vi "Execute.vi"(8 "error in (no error)":errorcluster, 9 "write enable":bool=TRUE, 10 "stop":bool, 11 "MB_TCP in":refnum<class "MB_TCP.lvclass">) -> (0 "error out":errorcluster, 2 "stopped":bool, 3 "MB_TCP out":refnum<class "MB_TCP.lvclass">)   [LabVIEW 2021, in "MB_TCP.lvclass"]
uses:
  MB_TCP.lvclass
  MB_TCP_State.ctl
  MB_TCP.lvclass/MB_TCP.ctl
  NI_modbus_upd/TCP/TCP.lvclass/TCP.ctl
  ICPCON Registers/MB ICPCON Registers Write DO.vi
  ICPCON Registers/MB ICPCON Registers Write IR.vi
  ICPCON Registers/MB ICPCON Registers Write DI.vi
  ICPCON Registers/MB ICPCON Registers Write OR.vi
  NI_modbus_upd/TCP/Accessors/Address/Write Address.vi
  NI_modbus_upd/TCP/Accessors/Port/Write Port.vi
  NI_modbus_upd/TCP/Accessors/connect timeout/Write timeouts.vi
  ICPCON Param/MB ICPCON Param Read timeout.vi
  Eth Status/Eth Status Read Error.vi
  Timer Delay/unix time 1ms.vi
  Eth Status/Eth Status.lvlib
  ICPCON Registers/ICPCON Registers.lvlib
  Timer Delay/Timers.lvlib
  ICPCON Param/ICPCON_Param.lvlib
panel:
  out "MB_TCP_State":T1=enum."requests"
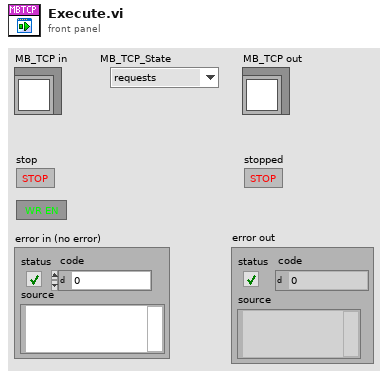
[diagram p1: front panel]
types:
  T1 = typedef "MB_TCP.lvclass/MB_TCP_State.ctl" = enum8{"initialization", "redefine", "standby", "connect", "wait to reconnect", "wait to reset timeout", "configure", "requests", "close connection", "stop"}
  T2 = typedef "ICPCON_Param.lvlib/ICPCON Param.ctl" = cluster{"IP addr":refnum<data-value>, "MVIName":refnum<data-value>, "timeouts":refnum<data-value>, "modified":refnum<data-value>}
  T3 = typedef "ICPCON Registers.lvlib/ICPCON Data.ctl" = cluster{"UTF":refnum<data-value>, "DI":refnum<data-value>, "DW":refnum<data-value>, "DO":refnum<data-value>, "IR":refnum<data-value>, "WR":refnum<data-value>, "OR":refnum<data-value>, "modified":refnum<data-value>}
  T4 = typedef "Eth Status.lvlib/Status.ctl" = cluster{"Set_states":refnum<queue>[], "WrEn":refnum<data-value>, "errors":refnum<data-value>, "connect":refnum<data-value>, "state":refnum<data-value>}
  T5 = typedef "MB_TCP.lvclass/MB timeouts.ctl" = cluster{"reconn_timeout":i32, "N attempt max":i32, "t_reset_TTL":i32, "period":i32}
  T6 = cluster{"Remote IP Address":string, "Remote Port":u16}
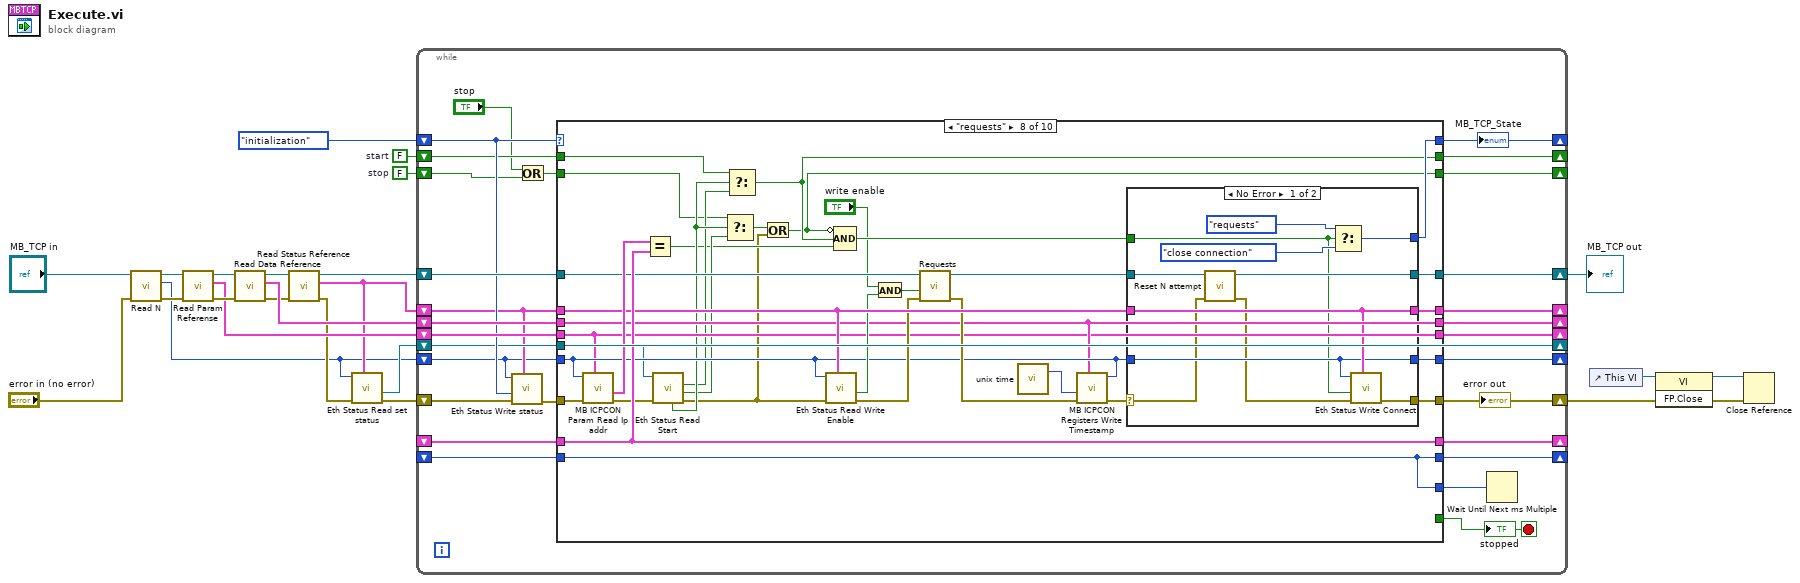
[diagram p0: block diagram]
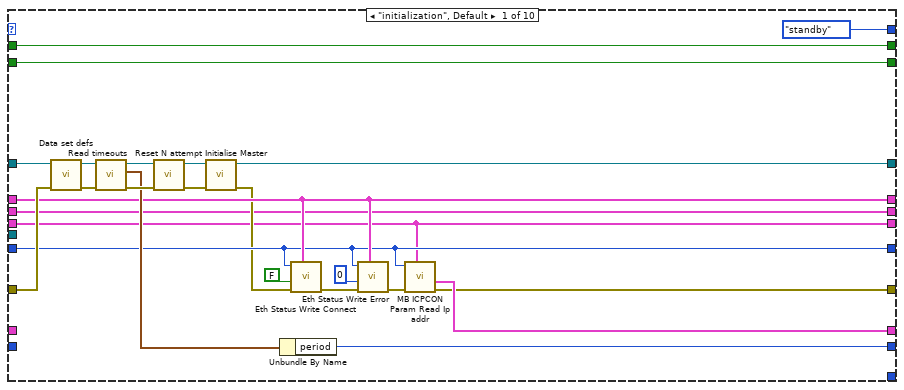
[diagram p2: hidden frame]
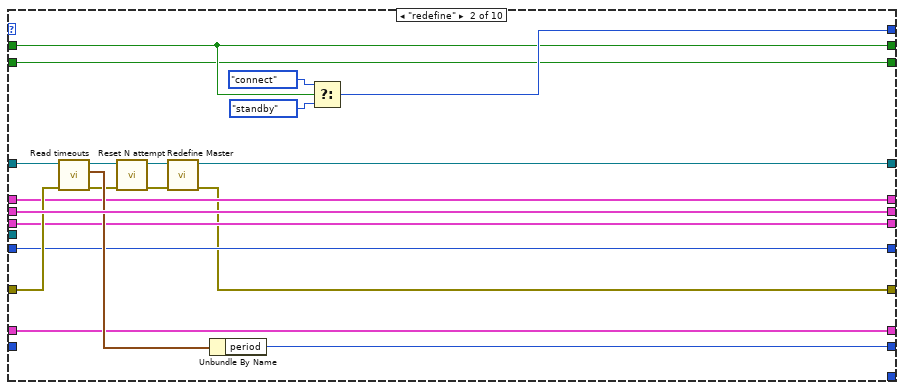
[diagram p3: hidden frame]
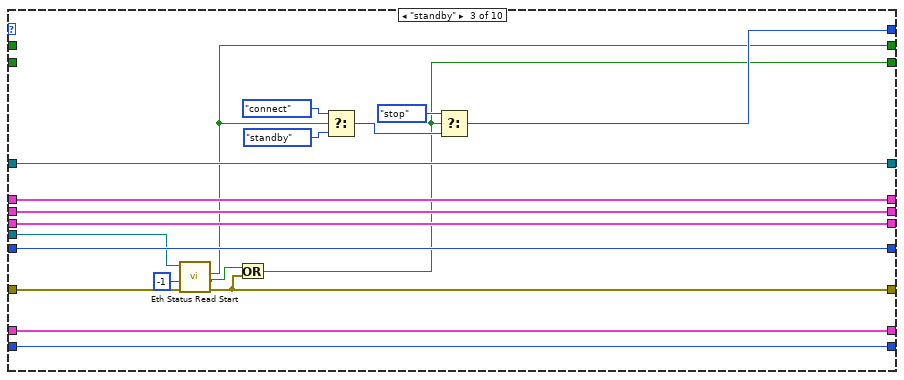
[diagram p4: hidden frame]
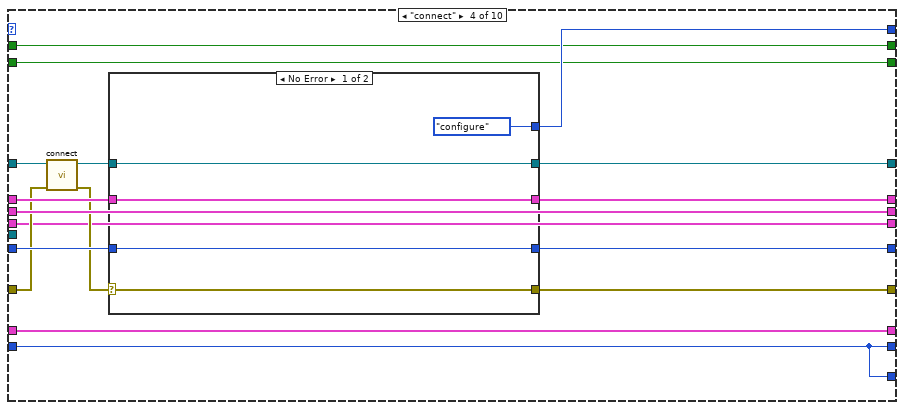
[diagram p5: hidden frame]
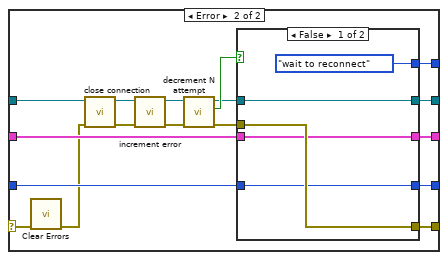
[diagram p6: hidden frame]
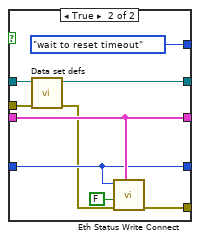
[diagram p7: hidden frame]
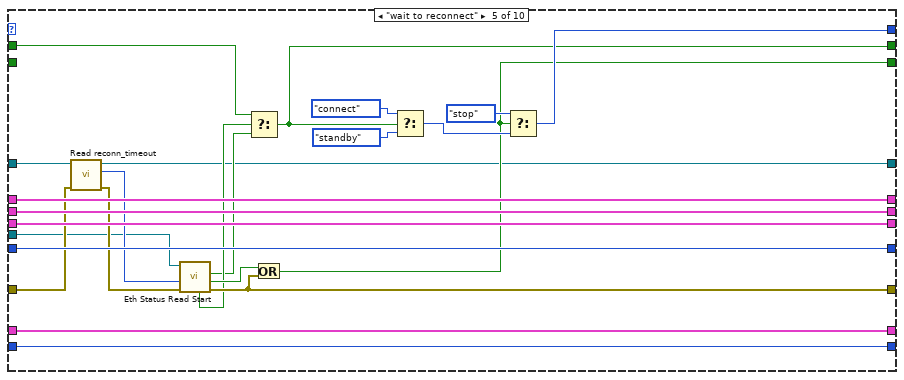
[diagram p8: hidden frame]
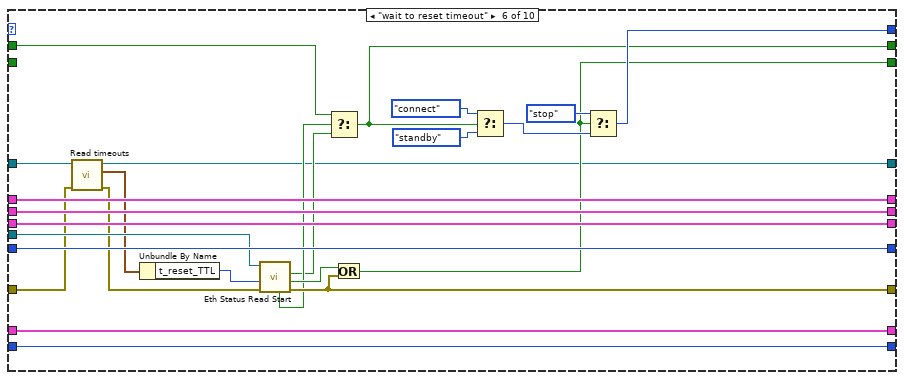
[diagram p9: hidden frame]
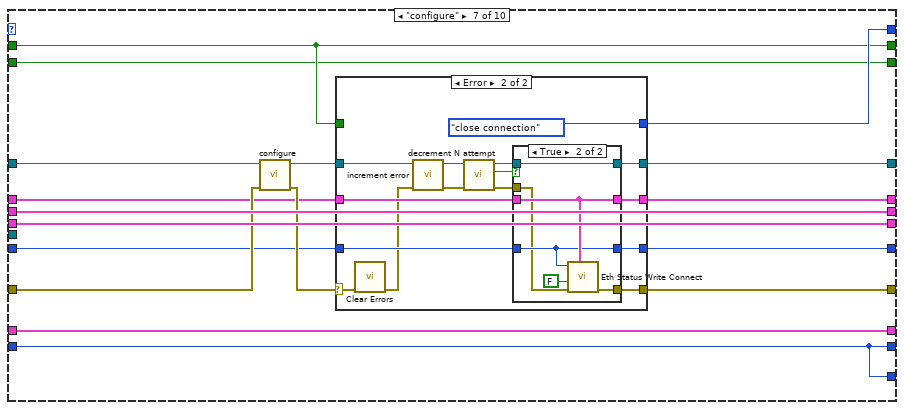
[diagram p10: hidden frame]
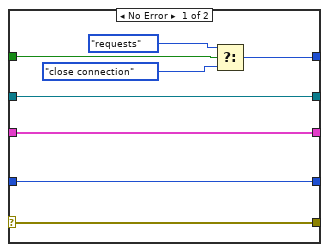
[diagram p11: hidden frame]
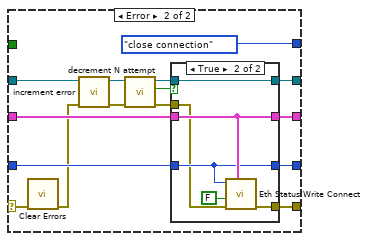
[diagram p13: hidden frame]
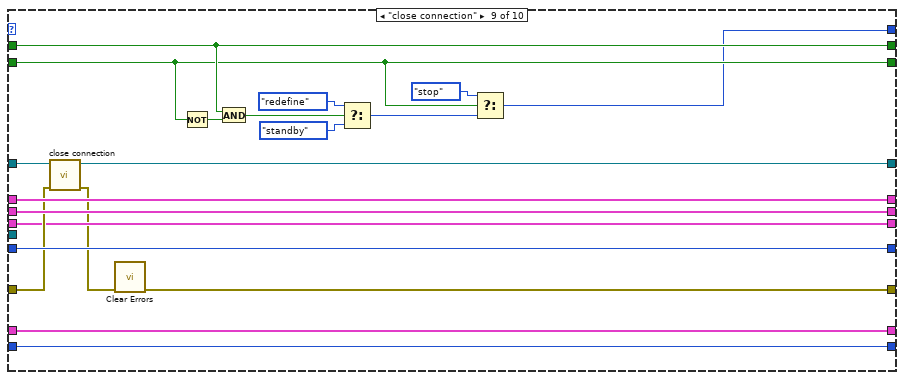
[diagram p15: hidden frame]
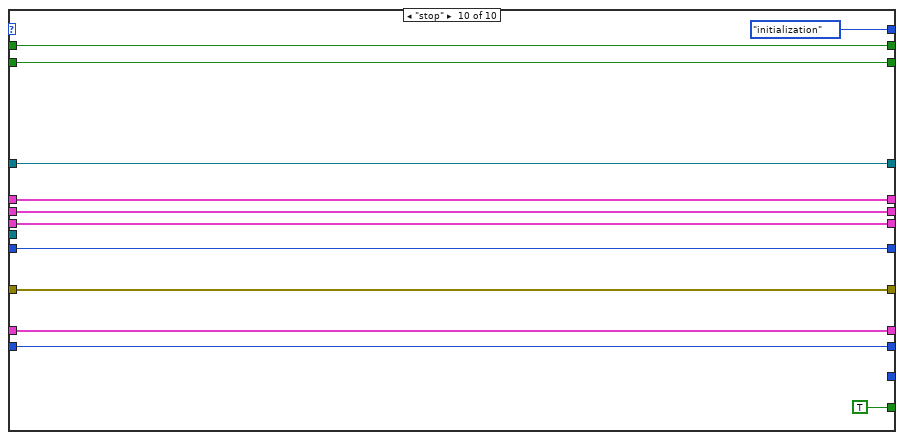
[diagram p16: hidden frame]
diagram:
  w1 = FALSE  # start
  w2 = FALSE  # stop
  n1 = call "Read N.vi"("error in (no error)"="error in (no error)", "MB_TCP in"="MB_TCP in") -> ("error out"=w16:errorcluster, "N"=w3:i32, "MB_TCP out"=w15:refnum<class "MB_TCP.lvclass">)  [unwired: 7 in]
  n2 = call "Read Param Referense.vi"("error in (no error)"=w16, "MB_TCP in"=w15) -> ("error out"=w13:errorcluster, "Param Referense"=w12:T2, "MB_TCP out"=w14:refnum<class "MB_TCP.lvclass">)  [unwired: 7 in]
  n3 = call "Read Data Reference.vi"("error in (no error)"=w13, "MB_TCP in"=w14) -> ("error out"=w17:errorcluster, "Data"=w20:T3, "MB_TCP out"=w18:refnum<class "MB_TCP.lvclass">)  [unwired: 7 in]
  n4 = call "Read Status Reference.vi"("error in (no error)"=w17, "MB_TCP in"=w18) -> ("error out"=w7:errorcluster, "Status"=w5:T4, "MB_TCP out"=w21:refnum<class "MB_TCP.lvclass">)  [unwired: 7 in]
  n5 = call "Eth Status Read set status.vi"("Status Reference"=w5, "error in (no error)"=w7, "N"=w3) -> ("error out"=w6:errorcluster, "set state"=w4:refnum<queue>)  [unwired: 7 in]
  n6 = while {
    shift-right: [w30] -> _
    shift-left: w2 -> [w28]
    shift-right: [w51] -> _
    shift-left: _ -> [w50]
    shift-right: [w49] -> _
    shift-left: w20 -> [w48]
    shift-right: [w32] -> w23
    shift-left: w21 -> [w44]
    shift-right: [w46] -> _
    shift-left: MB_TCP_State."initialization" ("MB_TCP_State") -> [w37]
    shift-right: [w38] -> _
    shift-left: w5 -> [w25]
    shift-right: [w39] -> _
    shift-left: w3 -> [w24]
    shift-right: [w36] -> w10
    shift-left: w6 -> [w27]
    shift-right: [w41] -> _
    shift-left: _ -> [w45]
    shift-right: [w42] -> _
    shift-left: w12 -> [w43]
    shift-right: [w34] -> _
    shift-left: w4 -> [w34]
    shift-right: [w31] -> _
    shift-left: w1 -> [w35]
    stop <- w47 stop-if-true
    n7 = call "Eth Status Write status.vi"("Status Reference"=w25, "error in (no error)"=w27, "status"=w37, "N"=w24) -> ("error out"=w26:errorcluster)  [unwired: 7 in]
    n8 = Or(x="stop", y=w28) -> (x .or. y?=w33:bool)
    n9 = case shown="\"requests\"" w37 {
      tunnel: w35 -> [w53 w78 _ w118 w180 w205 w219 w276 w343 w360]
      tunnel: w33 -> [w52 w77 _ w117 _ _ w218 w273 w341 w359]
      tunnel: [_ _ _ _ _ _ _ _ _ TRUE] -> w47
      tunnel: [w62 w80 w107 w119 w188 w213 w234 w301 w348 w362] -> w51
      tunnel: w50 -> [_ w80 w107 w119 w188 w213 w234 w301 w348 w362]
      tunnel: [w55 w96 w115 w132 w192 w217 w230 w283 w358 w370] -> w49
      tunnel: w48 -> [w55 w96 w115 w132 w192 w217 w230 w283 w358 w370]
      tunnel: w44 -> [w73 w92 w112 w123 w173 w198 w227 w291 w352 w363]
      tunnel: [w56 w82 w112 w131 w174 w197 w233 w297 w350 w363] -> w32
      tunnel: w26 -> [w74 w91 w103 w124 w171 w196 w224 w280 w351 w367]
      tunnel: [MB_TCP_State."standby" ("MB_TCP_State") w93 w109 w130 w177 w202 w232 w296 w339 MB_TCP_State."initialization" ("MB_TCP_State")] -> w46
      tunnel: [w64 w86 w105 w129 w191 w216 w222 w295 w355 w369] -> w38
      tunnel: [w63 w85 w104 w125 w190 w215 w220 w294 w354 w368] -> w39
      tunnel: w25 -> [w64 w86 w105 w128 w191 w216 w223 w292 w355 w369]
      tunnel: w24 -> [w63 w85 w104 w126 w190 w215 w221 w284 w354 w368]
      tunnel: [w60 w79 w102 w127 w181 w206 w231 w293 w346 w367] -> w36
      tunnel: [w75 w89 w106 w116 w187 w212 w228 w281 w353 w366] -> w41
      tunnel: w45 -> [_ _ w106 w116 w187 w212 w228 w281 w353 w366]
      tunnel: w43 -> [w54 w81 w111 w120 w189 w214 w229 w282 w349 w365]
      tunnel: [w54 w81 w111 w120 w189 w214 w229 w282 w349 w365] -> w42
      tunnel: [_ _ _ w116 _ _ w228 w281 _ _] -> w40
      tunnel: [w53 w78 w98 w118 w175 w200 w219 w271 w343 w360] -> w31
      tunnel: [w52 w77 w97 w117 w176 w201 w218 w270 w341 w359] -> w30
      tunnel: w34 -> [_ _ w101 _ w169 w199 _ w278 _ _]
      frame "initialization", Default {
        n10 = call "Data set defs.vi"("error in (no error)"=w74, "MB_TCP in"=w73) -> ("error out"=w61:errorcluster, "MB_TCP out"=w67:refnum<class "MB_TCP.lvclass">)  [unwired: 8 in]
        n11 = call "Read timeouts.vi"("error in (no error)"=w61, "MB_TCP in"=w67) -> ("error out"=w72:errorcluster, "MB timeouts"=w65:T5, "MB_TCP out"=w66:refnum<class "MB_TCP.lvclass">)  [unwired: 7 in]
        n12 = call "Reset N attempt.vi"("error in (no error)"=w72, "MB_TCP in"=w66) -> ("error out"=w58:errorcluster, "MB_TCP out"=w59:refnum<class "MB_TCP.lvclass">)  [unwired: 8 in]
        n13 = call "Initialise Master.vi"("error in (no error)"=w58, "MB_TCP in"=w59) -> ("error out"=w57:errorcluster, "MB_TCP out"=w56:refnum<class "MB_TCP.lvclass">)  [unwired: 8 in]
        n14 = Unbundle By Name(w65) -> ("period"=w75:i32)
        n15 = call "Eth Status Write Connect.vi"("Status Reference"=w64, "error in (no error)"=w57, "Connect"=FALSE ("connect"), "N"=w63) -> ("error out"=w69:errorcluster)  [unwired: 7 in]
        n16 = call "Eth Status Write Error.vi"("Status Reference"=w64, "error in (no error)"=w69, "Errors"=0 ("N attempt max"), "N"=w63) -> ("error out"=w68:errorcluster)  [unwired: 7 in]
        n17 = call "MB ICPCON Param Read Ip addr.vi"("Param Reference"=w54, "error in (no error)"=w68, "N"=w63) -> ("error out"=w60:errorcluster, "IP address"=w62:T6)  [unwired: 7 in]
      }
      frame "redefine" {
        n18 = call "Read timeouts.vi"("error in (no error)"=w91, "MB_TCP in"=w92) -> ("error out"=w88:errorcluster, "MB timeouts"=w90:T5, "MB_TCP out"=w87:refnum<class "MB_TCP.lvclass">)  [unwired: 7 in]
        n19 = call "Reset N attempt.vi"("error in (no error)"=w88, "MB_TCP in"=w87) -> ("error out"=w83:errorcluster, "MB_TCP out"=w84:refnum<class "MB_TCP.lvclass">)  [unwired: 8 in]
        n20 = call "Redefine Master.vi"("error in (no error)"=w83, "MB_TCP in"=w84) -> ("error out"=w79:errorcluster, "MB_TCP out"=w82:refnum<class "MB_TCP.lvclass">)  [unwired: 8 in]
        n21 = Unbundle By Name(w90) -> ("period"=w89:i32)
        n22 = Select(t=MB_TCP_State."connect" ("MB_TCP_State"), s=w78, f=MB_TCP_State."standby" ("MB_TCP_State")) -> (s? t:f=w93:T1)
      }
      frame "standby" {
        n23 = call "Eth Status Read Start.vi"("error in (no error)"=w103, "timeout (0)"=-1, "Set_state"=w101) -> ("error out"=w102:errorcluster, "Stop"=w99:bool, "Start"=w98:bool)  [unwired: 4 in, 2 out]
        n24 = Or(x=w99, y=w102) -> (x .or. y?=w97:bool)
        n25 = Select(t=MB_TCP_State."connect" ("MB_TCP_State"), s=w98, f=MB_TCP_State."standby" ("MB_TCP_State")) -> (s? t:f=w108:T1)
        n26 = Select(t=MB_TCP_State."stop" ("MB_TCP_State"), s=w97, f=w108) -> (s? t:f=w109:T1)
      }
      frame "connect" {
        n27 = call-dynamic "connect.vi"("error in (no error)"=w124, "MB_TCP in"=w123) -> ("error out"=w121:errorcluster, "MB_TCP out"=w122:refnum<class "MB_TCP.lvclass">)  [unwired: 8 in]
        n28 = case shown="No Error" w121 {
          selector: w121 -> [w135 w142]
          tunnel: w122 -> [w136 w143]
          tunnel: [MB_TCP_State."configure" ("MB_TCP_State") w152] -> w130
          tunnel: [w136 w147] -> w131
          tunnel: [w135 w146] -> w127
          tunnel: w128 -> [w134 w148]
          tunnel: w126 -> [w133 w149]
          tunnel: [w134 w151] -> w129
          tunnel: [w133 w150] -> w125
          frame No Error {
          }
          frame Error {
            n29 = call <vilib>:"Clear Errors.vi"("error in (no error)"=w142) -> ("error out"=w141:errorcluster)  [unwired: 5 in, 1 out]
            n30 = call-dynamic "close connection.vi"("error in (no error)"=w141, "MB_TCP in"=w143) -> ("error out"=w144:errorcluster, "MB_TCP out"=w145:refnum<class "MB_TCP.lvclass">)  [unwired: 8 in]
            n31 = call "increment error.vi"("error in (no error)"=w144, "MB_TCP in"=w145) -> ("error out"=w140:errorcluster, "MB_TCP out"=w154:refnum<class "MB_TCP.lvclass">)  [unwired: 7 in, 1 out]
            n32 = call "decrement N attempt.vi"("error in (no error)"=w140, "MB_TCP in"=w154) -> ("error out"=w138:errorcluster, "=0"=w153:bool, "MB_TCP out"=w139:refnum<class "MB_TCP.lvclass">)  [unwired: 7 in]
            n33 = case shown="False" w153 {
              tunnel: [MB_TCP_State."wait to reconnect" ("MB_TCP_State") MB_TCP_State."wait to reset timeout" ("MB_TCP_State")] -> w152
              tunnel: w139 -> [w158 w163]
              tunnel: [w158 w161] -> w147
              tunnel: w138 -> [w157 w162]
              tunnel: [w157 w166] -> w146
              tunnel: w148 -> [w156 w165]
              tunnel: w149 -> [w155 w164]
              tunnel: [w156 w165] -> w151
              tunnel: [w155 w164] -> w150
              frame False {
              }
              frame True {
                n34 = call "Data set defs.vi"("error in (no error)"=w162, "MB_TCP in"=w163) -> ("error out"=w160:errorcluster, "MB_TCP out"=w161:refnum<class "MB_TCP.lvclass">)  [unwired: 8 in]
                n35 = call "Eth Status Write Connect.vi"("Status Reference"=w165, "error in (no error)"=w160, "Connect"=FALSE ("f"), "N"=w164) -> ("error out"=w166:errorcluster)  [unwired: 7 in]
              }
            }
          }
        }
      }
      frame "wait to reconnect" {
        n36 = call "Read reconn_timeout.vi"("error in (no error)"=w171, "MB_TCP in"=w173) -> ("error out"=w172:errorcluster, "reconn_timeout"=w170:i32, "MB_TCP out"=w174:refnum<class "MB_TCP.lvclass">)  [unwired: 7 in]
        n37 = call "Eth Status Read Start.vi"("error in (no error)"=w172, "timeout (0)"=w170, "Set_state"=w169) -> ("error out"=w181:errorcluster, "Stop"=w182:bool, "Start"=w178:bool, "timed out?"=w179:bool)  [unwired: 4 in, 1 out]
        n38 = Select(t=w180, s=w179, f=w178) -> (s? t:f=w175:bool)
        n39 = Or(x=w182, y=w181) -> (x .or. y?=w176:bool)
        n40 = Select(t=MB_TCP_State."connect" ("MB_TCP_State"), s=w175, f=MB_TCP_State."standby" ("MB_TCP_State")) -> (s? t:f=w183:T1)
        n41 = Select(t=MB_TCP_State."stop" ("MB_TCP_State"), s=w176, f=w183) -> (s? t:f=w177:T1)
      }
      frame "wait to reset timeout" {
        n42 = call "Read timeouts.vi"("error in (no error)"=w196, "MB_TCP in"=w198) -> ("error out"=w195:errorcluster, "MB timeouts"=w194:T5, "MB_TCP out"=w197:refnum<class "MB_TCP.lvclass">)  [unwired: 7 in]
        n43 = Unbundle By Name(w194) -> ("t_reset_TTL"=w193:i32)
        n44 = call "Eth Status Read Start.vi"("error in (no error)"=w195, "timeout (0)"=w193, "Set_state"=w199) -> ("error out"=w206:errorcluster, "Stop"=w207:bool, "Start"=w203:bool, "timed out?"=w204:bool)  [unwired: 4 in, 1 out]
        n45 = Select(t=w205, s=w204, f=w203) -> (s? t:f=w200:bool)
        n46 = Or(x=w207, y=w206) -> (x .or. y?=w201:bool)
        n47 = Select(t=MB_TCP_State."connect" ("MB_TCP_State"), s=w200, f=MB_TCP_State."standby" ("MB_TCP_State")) -> (s? t:f=w208:T1)
        n48 = Select(t=MB_TCP_State."stop" ("MB_TCP_State"), s=w201, f=w208) -> (s? t:f=w202:T1)
      }
      frame "configure" {
        n49 = call-dynamic "configure.vi"("error in (no error)"=w224, "MB_TCP in"=w227) -> ("error out"=w225:errorcluster, "MB_TCP out"=w226:refnum<class "MB_TCP.lvclass">)  [unwired: 8 in]
        n50 = case shown="Error" w225 {
          selector: w225 -> [w237 w256]
          tunnel: [w242 MB_TCP_State."close connection" ("MB_TCP_State")] -> w232
          tunnel: w219 -> [w239 _]
          tunnel: [w237 w247] -> w231
          tunnel: w226 -> [w238 w244]
          tunnel: [w238 w248] -> w233
          tunnel: w223 -> [w236 w250]
          tunnel: [w236 w249] -> w222
          tunnel: w221 -> [w235 w246]
          tunnel: [w235 w245] -> w220
          frame No Error {
            n51 = Select(t=MB_TCP_State."requests" ("MB_TCP_State"), s=w239, f=MB_TCP_State."close connection" ("MB_TCP_State")) -> (s? t:f=w242:T1)
          }
          frame Error {
            n52 = call <vilib>:"Clear Errors.vi"("error in (no error)"=w256) -> ("error out"=w243:errorcluster)  [unwired: 5 in, 1 out]
            n53 = call "increment error.vi"("error in (no error)"=w243, "MB_TCP in"=w244) -> ("error out"=w252:errorcluster, "MB_TCP out"=w251:refnum<class "MB_TCP.lvclass">)  [unwired: 7 in, 1 out]
            n54 = call "decrement N attempt.vi"("error in (no error)"=w252, "MB_TCP in"=w251) -> ("error out"=w253:errorcluster, "=0"=w255:bool, "MB_TCP out"=w254:refnum<class "MB_TCP.lvclass">)  [unwired: 7 in]
            n55 = case shown="True" w255 {
              tunnel: w254 -> [w261 w263]
              tunnel: [w261 w263] -> w248
              tunnel: w253 -> [w260 w262]
              tunnel: [w260 w266] -> w247
              tunnel: w250 -> [w259 w265]
              tunnel: w246 -> [w258 w264]
              tunnel: [w259 w265] -> w249
              tunnel: [w258 w264] -> w245
              frame False {
              }
              frame True {
                n56 = call "Eth Status Write Connect.vi"("Status Reference"=w265, "error in (no error)"=w262, "Connect"=FALSE ("f"), "N"=w264) -> ("error out"=w266:errorcluster)  [unwired: 7 in]
              }
            }
          }
        }
      }
      frame "requests" {
        n57 = call "MB ICPCON Param Read Ip addr.vi"("Param Reference"=w282, "error in (no error)"=w280, "N"=w284) -> ("error out"=w279:errorcluster, "IP address"=w298:T6)  [unwired: 7 in]
        n58 = Equal?(x=w298, y=w301) -> (x = y?=w272:bool)
        n59 = call "Eth Status Read Start.vi"("error in (no error)"=w279, "Set_state"=w278) -> ("error out"=w268:errorcluster, "Stop"=w274:bool, "Start"=w275:bool, "timed out?"=w277:bool)  [unwired: 5 in, 1 out]
        n60 = Select(t=w273, s=w277, f=w274) -> (s? t:f=w269:bool)
        n61 = Select(t=w276, s=w277, f=w275) -> (s? t:f=w271:bool)
        n62 = Or(x=w269, y=w268) -> (x .or. y?=w270:bool)
        n63 = call "Eth Status Read Write Enable.vi"("Status Reference"=w292, "error in (no error)"=w268, "N"=w284) -> ("error out"=w289:errorcluster, "Write Enable"=w287:bool)  [unwired: 7 in]
        n64 = Compound Arithmetic op=AND(invert w270, w271, w272) -> (w302:bool)
        n65 = And(x="write enable", y=w287) -> (x .and. y?=w285:bool)
        n66 = call-dynamic "Requests.vi"("error in (no error)"=w289, "write enable"=w285, "MB_TCP in"=w291) -> ("error out"=w288:errorcluster, "MB_TCP out"=w290:refnum<class "MB_TCP.lvclass">)  [unwired: 7 in]
        n67 = call-poly "unix time.vi"() -> ("unix time (ms)"=w299:u64)  [unwired: 2 in, 1 out]
        n68 = call "MB ICPCON Registers Write Timestamp.vi"("Data Reference"=w283, "error in (no error)"=w288, "UTF"=w299, "N"=w284) -> ("error out"=w300:errorcluster)  [unwired: 7 in]
        n69 = case shown="No Error" w300 {
          selector: w300 -> [w307 w327]
          tunnel: [w313 MB_TCP_State."close connection" ("MB_TCP_State")] -> w296
          tunnel: w302 -> [w303 _]
          tunnel: [w306 w318] -> w293
          tunnel: w292 -> [w309 w325]
          tunnel: w290 -> [w310 w315]
          tunnel: [w304 w319] -> w297
          tunnel: [w309 w323] -> w295
          tunnel: w284 -> [w308 w324]
          tunnel: [w308 w322] -> w294
          frame No Error {
            n70 = call "Reset N attempt.vi"("error in (no error)"=w307, "MB_TCP in"=w310) -> ("error out"=w305:errorcluster, "MB_TCP out"=w304:refnum<class "MB_TCP.lvclass">)  [unwired: 8 in]
            n71 = Select(t=MB_TCP_State."requests" ("MB_TCP_State"), s=w303, f=MB_TCP_State."close connection" ("MB_TCP_State")) -> (s? t:f=w313:T1)
            n72 = call "Eth Status Write Connect.vi"("Status Reference"=w309, "error in (no error)"=w305, "Connect"=w303, "N"=w308) -> ("error out"=w306:errorcluster)  [unwired: 7 in]
          }
          frame Error {
            n73 = call <vilib>:"Clear Errors.vi"("error in (no error)"=w327) -> ("error out"=w314:errorcluster)  [unwired: 5 in, 1 out]
            n74 = call "increment error.vi"("error in (no error)"=w314, "MB_TCP in"=w315) -> ("error out"=w316:errorcluster, "MB_TCP out"=w321:refnum<class "MB_TCP.lvclass">)  [unwired: 7 in, 1 out]
            n75 = call "decrement N attempt.vi"("error in (no error)"=w316, "MB_TCP in"=w321) -> ("error out"=w317:errorcluster, "=0"=w326:bool, "MB_TCP out"=w320:refnum<class "MB_TCP.lvclass">)  [unwired: 7 in]
            n76 = case shown="True" w326 {
              tunnel: w320 -> [w332 w334]
              tunnel: [w332 w334] -> w319
              tunnel: w317 -> [w331 w333]
              tunnel: [w331 w337] -> w318
              tunnel: w325 -> [w330 w336]
              tunnel: w324 -> [w329 w335]
              tunnel: [w330 w336] -> w323
              tunnel: [w329 w335] -> w322
              frame False {
              }
              frame True {
                n77 = call "Eth Status Write Connect.vi"("Status Reference"=w336, "error in (no error)"=w333, "Connect"=FALSE ("f"), "N"=w335) -> ("error out"=w337:errorcluster)  [unwired: 7 in]
              }
            }
          }
        }
      }
      frame "close connection" {
        n78 = call-dynamic "close connection.vi"("error in (no error)"=w351, "MB_TCP in"=w352) -> ("error out"=w347:errorcluster, "MB_TCP out"=w350:refnum<class "MB_TCP.lvclass">)  [unwired: 8 in]
        n79 = call <vilib>:"Clear Errors.vi"("error in (no error)"=w347) -> ("error out"=w346:errorcluster)  [unwired: 5 in, 1 out]
        n80 = Not(x=w341) -> (.not. x?=w345:bool)
        n81 = And(x=w343, y=w345) -> (x .and. y?=w344:bool)
        n82 = Select(t=MB_TCP_State."redefine" ("MB_TCP_State"), s=w344, f=MB_TCP_State."standby" ("MB_TCP_State")) -> (s? t:f=w340:T1)
        n83 = Select(t=MB_TCP_State."stop" ("MB_TCP_State"), s=w341, f=w340) -> (s? t:f=w339:T1)
      }
      frame "stop" {
      }
    }
    "stopped" <- w47
    "error out" <- w36
    "MB_TCP_State" <- w46
    n84 = Wait Until Next ms Multiple(millisecond multiple=w40) -> ()  [unwired: 1 out]
  }
  "MB_TCP out" <- w23
  n85 = control-ref of="This VI"() -> (w9:refnum<vi>)
  n86 = invoke class="VI" method="FP.Close"(reference=w9) -> (reference out=w8:refnum<vi>)  [unwired: 2 in, 2 out]
  n87 = Close Reference(reference=w8, error in (no error)=w10) -> ()  [unwired: 1 out]
